vi "VI Tree.vi"   [LabVIEW 2016, in "eec EST 300.lvlib"]
doc: "The VI Tree displays all the user-callable VIs of the instrument driver in an organized table."
uses:
  <instrlib>/eec EST 300/eec EST 300.lvlib
panel:
  # "Please see diagram for EEC EST 300 Driver VI Tree"
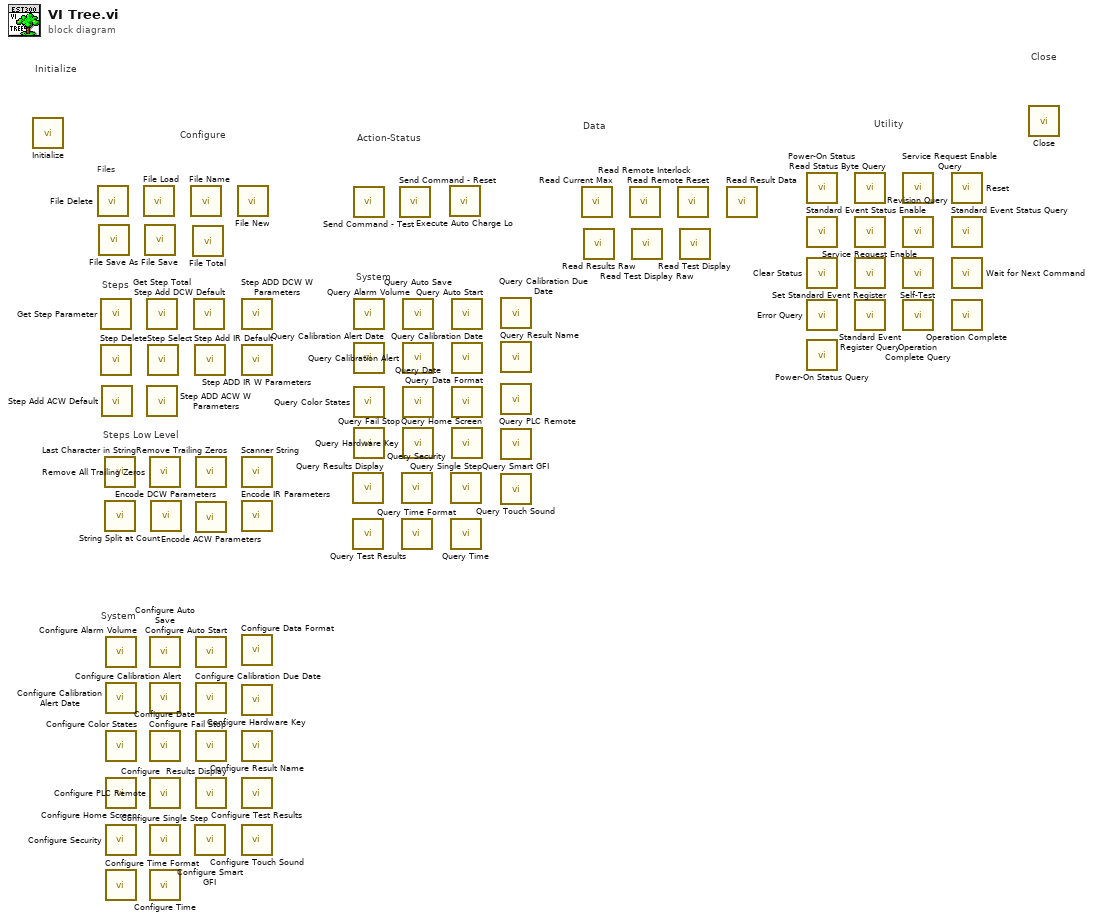
[diagram p0: block diagram]
diagram:
  # "Steps Low Level"
  # "System"
  # "Data"
  # "System"
  # "Steps"
  # "Files"
  # "Configure"
  # "Utility"
  # "Action-Status"
  # "Close"
  # "Initialize"
  n1 = call <instrlib>:"Initialize.vi"() -> ()  [unwired: 13 in, 3 out]
  n2 = call <instrlib>:"File Delete.vi"() -> ()  [unwired: 14 in, 2 out]
  n3 = call <instrlib>:"File Save As.vi"() -> ()  [unwired: 14 in, 2 out]
  n4 = call <instrlib>:"Get Step Parameter.vi"() -> ()  [unwired: 13 in, 3 out]
  n5 = call <instrlib>:"Step Delete.vi"() -> ()  [unwired: 14 in, 2 out]
  n6 = call <instrlib>:"Step Add ACW Default.vi"() -> ()  [unwired: 10 in, 2 out]
  n7 = call <instrlib>:"Last Character in String.vi"() -> ()  [unwired: 1 in, 2 out]
  n8 = call <instrlib>:"String Split at Count.vi"() -> ()  [unwired: 2 in, 2 out]
  n9 = call <instrlib>:"Configure Alarm Volume.vi"() -> ()  [unwired: 10 in, 2 out]
  n10 = call <instrlib>:"Configure Calibration Alert Date.vi"() -> ()  [unwired: 14 in, 2 out]
  n11 = call <instrlib>:"Configure Color States.vi"() -> ()  [unwired: 10 in, 2 out]
  n12 = call <instrlib>:"Configure Home Screen.vi"() -> ()  [unwired: 10 in, 2 out]
  n13 = call <instrlib>:"Configure Security.vi"() -> ()  [unwired: 14 in, 2 out]
  n14 = call <instrlib>:"Configure Time Format.vi"() -> ()  [unwired: 10 in, 2 out]
  n15 = call <instrlib>:"File Load.vi"() -> ()  [unwired: 14 in, 2 out]
  n16 = call <instrlib>:"File Save.vi"() -> ()  [unwired: 14 in, 2 out]
  n17 = call <instrlib>:"Get Step Total.vi"() -> ()  [unwired: 13 in, 3 out]
  n18 = call <instrlib>:"Step ADD ACW W Parameters.vi"() -> ()  [unwired: 14 in, 2 out]
  n19 = call <instrlib>:"Step Select.vi"() -> ()  [unwired: 14 in, 2 out]
  n20 = call <instrlib>:"Remove All Trailing Zeros.vi"() -> ()  [unwired: 1 in, 1 out]
  n21 = call <instrlib>:"Configure Auto Save.vi"() -> ()  [unwired: 14 in, 2 out]
  n22 = call <instrlib>:"Configure Calibration Alert.vi"() -> ()  [unwired: 10 in, 2 out]
  n23 = call <instrlib>:"Configure Date.vi"() -> ()  [unwired: 14 in, 2 out]
  n24 = call <instrlib>:"Configure PLC Remote.vi"() -> ()  [unwired: 10 in, 2 out]
  n25 = call <instrlib>:"Configure Single Step.vi"() -> ()  [unwired: 14 in, 2 out]
  n26 = call <instrlib>:"Configure Time.vi"() -> ()  [unwired: 14 in, 2 out]
  n27 = call <instrlib>:"Encode DCW Parameters.vi"() -> ()  [unwired: 9 in, 3 out]
  n28 = call <instrlib>:"File Name.vi"() -> ()  [unwired: 13 in, 3 out]
  n29 = call <instrlib>:"File Total.vi"() -> ()  [unwired: 13 in, 3 out]
  n30 = call <instrlib>:"Step Add DCW Default.vi"() -> ()  [unwired: 10 in, 2 out]
  n31 = call <instrlib>:"Step Add IR Default.vi"() -> ()  [unwired: 10 in, 2 out]
  n32 = call <instrlib>:"Configure Smart GFI.vi"() -> ()  [unwired: 14 in, 2 out]
  n33 = call <instrlib>:"Remove Trailing Zeros.vi"() -> ()  [unwired: 1 in, 1 out]
  n34 = call <instrlib>:"Encode ACW Parameters.vi"() -> ()  [unwired: 9 in, 3 out]
  n35 = call <instrlib>:"Configure Auto Start.vi"() -> ()  [unwired: 14 in, 2 out]
  n36 = call <instrlib>:"Configure Calibration Due Date.vi"() -> ()  [unwired: 14 in, 2 out]
  n37 = call <instrlib>:"Configure Fail Stop.vi"() -> ()  [unwired: 14 in, 2 out]
  n38 = call <instrlib>:"Configure  Results Display.vi"() -> ()  [unwired: 10 in, 2 out]
  n39 = call <instrlib>:"File New.vi"() -> ()  [unwired: 14 in, 2 out]
  n40 = call <instrlib>:"Step ADD DCW W Parameters.vi"() -> ()  [unwired: 14 in, 2 out]
  n41 = call <instrlib>:"Step ADD IR W Parameters.vi"() -> ()  [unwired: 14 in, 2 out]
  n42 = call <instrlib>:"Scanner String.vi"() -> ()  [unwired: 2 in, 2 out]
  n43 = call <instrlib>:"Encode IR Parameters.vi"() -> ()  [unwired: 9 in, 3 out]
  n44 = call <instrlib>:"Configure Data Format.vi"() -> ()  [unwired: 10 in, 2 out]
  n45 = call <instrlib>:"Configure Hardware Key.vi"() -> ()  [unwired: 14 in, 2 out]
  n46 = call <instrlib>:"Configure Result Name.vi"() -> ()  [unwired: 10 in, 2 out]
  n47 = call <instrlib>:"Configure Test Results.vi"() -> ()  [unwired: 10 in, 2 out]
  n48 = call <instrlib>:"Configure Touch Sound.vi"() -> ()  [unwired: 14 in, 2 out]
  n49 = call <instrlib>:"Query Results Display.vi"() -> ()  [unwired: 9 in, 3 out]
  n50 = call <instrlib>:"Query Test Results.vi"() -> ()  [unwired: 9 in, 3 out]
  n51 = call <instrlib>:"Send Command - Test.vi"() -> ()  [unwired: 14 in, 2 out]
  n52 = call <instrlib>:"Query Alarm Volume.vi"() -> ()  [unwired: 9 in, 3 out]
  n53 = call <instrlib>:"Query Calibration Alert Date.vi"() -> ()  [unwired: 10 in, 6 out]
  n54 = call <instrlib>:"Query Color States.vi"() -> ()  [unwired: 9 in, 3 out]
  n55 = call <instrlib>:"Query Fail Stop.vi"() -> ()  [unwired: 9 in, 3 out]
  n56 = call <instrlib>:"Send Command - Reset.vi"() -> ()  [unwired: 14 in, 2 out]
  n57 = call <instrlib>:"Query Security.vi"() -> ()  [unwired: 9 in, 3 out]
  n58 = call <instrlib>:"Query Time Format.vi"() -> ()  [unwired: 9 in, 3 out]
  n59 = call <instrlib>:"Query Auto Save.vi"() -> ()  [unwired: 9 in, 3 out]
  n60 = call <instrlib>:"Query Calibration Alert.vi"() -> ()  [unwired: 9 in, 3 out]
  n61 = call <instrlib>:"Query Date.vi"() -> ()  [unwired: 10 in, 6 out]
  n62 = call <instrlib>:"Query Hardware Key.vi"() -> ()  [unwired: 9 in, 3 out]
  n63 = call <instrlib>:"Execute Auto Charge Lo.vi"() -> ()  [unwired: 14 in, 2 out]
  n64 = call <instrlib>:"Query Single Step.vi"() -> ()  [unwired: 9 in, 3 out]
  n65 = call <instrlib>:"Query Time.vi"() -> ()  [unwired: 8 in, 4 out]
  n66 = call <instrlib>:"Query Auto Start.vi"() -> ()  [unwired: 9 in, 3 out]
  n67 = call <instrlib>:"Query Calibration Date.vi"() -> ()  [unwired: 10 in, 6 out]
  n68 = call <instrlib>:"Query Data Format.vi"() -> ()  [unwired: 9 in, 3 out]
  n69 = call <instrlib>:"Query Home Screen.vi"() -> ()  [unwired: 9 in, 3 out]
  n70 = call <instrlib>:"Query Calibration Due Date.vi"() -> ()  [unwired: 10 in, 6 out]
  n71 = call <instrlib>:"Query Result Name.vi"() -> ()  [unwired: 9 in, 3 out]
  n72 = call <instrlib>:"Query PLC Remote.vi"() -> ()  [unwired: 9 in, 3 out]
  n73 = call <instrlib>:"Query Smart GFI.vi"() -> ()  [unwired: 9 in, 3 out]
  n74 = call <instrlib>:"Query Touch Sound.vi"() -> ()  [unwired: 9 in, 3 out]
  n75 = call <instrlib>:"Read Current Max.vi"() -> ()  [unwired: 13 in, 3 out]
  n76 = call <instrlib>:"Read Results Raw.vi"() -> ()  [unwired: 13 in, 3 out]
  n77 = call <instrlib>:"Read Remote Interlock.vi"() -> ()  [unwired: 13 in, 3 out]
  n78 = call <instrlib>:"Read Test Display Raw.vi"() -> ()  [unwired: 13 in, 3 out]
  n79 = call <instrlib>:"Read Remote Reset.vi"() -> ()  [unwired: 13 in, 3 out]
  n80 = call <instrlib>:"Read Test Display.vi"() -> ()  [unwired: 13 in, 3 out]
  n81 = call <instrlib>:"Read Result Data.vi"() -> ()  [unwired: 13 in, 3 out]
  n82 = call <instrlib>:"Power-On Status.vi"() -> ()  [unwired: 14 in, 2 out]
  n83 = call <instrlib>:"Standard Event Status Enable.vi"() -> ()  [unwired: 14 in, 2 out]
  n84 = call <instrlib>:"Clear Status.vi"() -> ()  [unwired: 14 in, 2 out]
  n85 = call <instrlib>:"Error Query.vi"() -> ()  [unwired: 12 in, 4 out]
  n86 = call <instrlib>:"Power-On Status Query.vi"() -> ()  [unwired: 13 in, 3 out]
  n87 = call <instrlib>:"Read Status Byte Query.vi"() -> ()  [unwired: 13 in, 3 out]
  n88 = call <instrlib>:"Service Request Enable.vi"() -> ()  [unwired: 14 in, 2 out]
  n89 = call <instrlib>:"Set Standard Event Register.vi"() -> ()  [unwired: 14 in, 2 out]
  n90 = call <instrlib>:"Standard Event Register Query.vi"() -> ()  [unwired: 13 in, 3 out]
  n91 = call <instrlib>:"Service Request Enable Query.vi"() -> ()  [unwired: 13 in, 3 out]
  n92 = call <instrlib>:"Revision Query.vi"() -> ()  [unwired: 11 in, 5 out]
  n93 = call <instrlib>:"Self-Test.vi"() -> ()  [unwired: 12 in, 4 out]
  n94 = call <instrlib>:"Operation Complete Query.vi"() -> ()  [unwired: 13 in, 3 out]
  n95 = call <instrlib>:"Reset.vi"() -> ()  [unwired: 14 in, 2 out]
  n96 = call <instrlib>:"Standard Event Status Query.vi"() -> ()  [unwired: 13 in, 3 out]
  n97 = call <instrlib>:"Wait for Next Command.vi"() -> ()  [unwired: 14 in, 2 out]
  n98 = call <instrlib>:"Operation Complete.vi"() -> ()  [unwired: 14 in, 2 out]
  n99 = call <instrlib>:"Close.vi"() -> ()  [unwired: 15 in, 1 out]
